vi "AddUniquePaths.vi"(8 "header files in":path[](array[path]), 10 "selected paths":path[](array[path])) -> (1 "appended array":path[](array[path]))   [LabVIEW 2016]
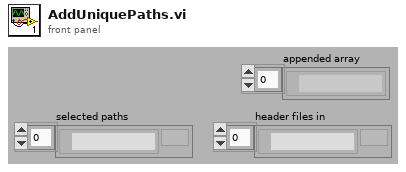
[diagram p1: front panel]
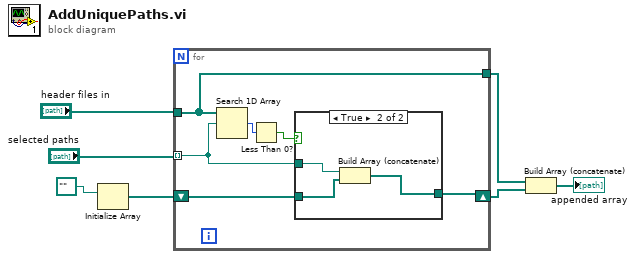
[diagram p0: block diagram]
diagram:
  n1 = Initialize Array(path "" ("element")) -> (w5:path[])  [unwired: 1 in]
  n2 = for {
    tunnel: "selected paths" -> [w11] mode=indexing
    tunnel: "header files in" -> [w8]
    shift-right: [w9] -> w2
    shift-left: w5 -> [w10]
    tunnel: [w8] -> w3
    n3 = Search 1D Array(1D array=w8, element=w11) -> (index of element=w13:i32)  [unwired: 1 in]
    n4 = Less Than 0?(x=w13) -> (x < 0?=w12:bool)
    n5 = case shown="True" w12 {
      tunnel: w11 -> [_ w17]
      tunnel: w10 -> [w14 w16]
      tunnel: [w14 w15] -> w9
      frame False {
      }
      frame True {
        n6 = Build Array (concatenate) "Build Array"(w17, w16) -> (w15:path[])
      }
    }
  }
  n7 = Build Array (concatenate)(w3, w2) -> (→"appended array":path[])
